vi "GetParamsVIS_K2182and6221.vi"(11 "KEITHLEY 2182 & KEITHLEY 6221_In":refnum<vi>) -> (0 "Params VIS K2182and6221_out":T2, 3 "KEITHLEY 2182 & KEITHLEY 6221_Out":refnum<vi>)   [LabVIEW 2013]
uses:
  TypeDef/EnumSelectedModeK2182and6221.ctl
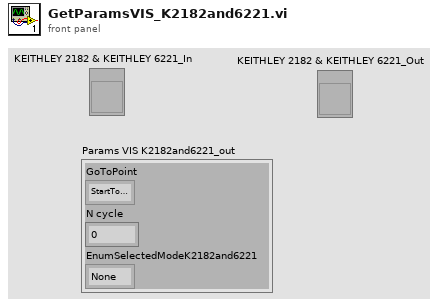
[diagram p1: front panel]
types:
  T1 = typedef "EnumSelectedModeK2182and6221.ctl" = enum16{"None", "K2182V", "K2182VI", "K2182VIS"}
  T2 = cluster{"GoToPoint":enum16{"StartToFront", "FrontToStart", "StartToBack", "BackToStart"}, "N cycle":i32, "EnumSelectedModeK2182and6221":T1}
  T3 = typedef "Keithly user program.lvlib/KE2182 -- Params.ctl" = cluster{"Auto Range?":bool, "Man / Selected\n       Range":enum16{"10mV", "100mV", "1V", "10V", "100V"}, "Enable Digital\n       Filter?":bool, "Filter Type":enum16{"Movin", "Repeat"}, "Filter Count":u32, "      Filter\nWindow (%)":dbl, "Enable Analog\n       Filter?":bool, "NPLCs":u32}
  T4 = typedef "Keithly user program.lvlib/KE622x -- Current Range.ctl" = cluster{"Auto Range?":bool, "Man / Selected\n        Range":enum16{"2nA", "20nA", "200nA", "2uA", "20uA", "200uA", "2mA", "20mA", "100mA"}}
  T5 = typedef "Keithly user program.lvlib/KE622x -- Current Level.ctl" = dbl
  T6 = typedef "Keithly user program.lvlib/KE622x -- Voltage Limit.ctl" = dbl
  T7 = typedef "Keithly user program.lvlib/KE6221 -- Output Response.ctl" = enum16{"Fast", "Slow"}
  T8 = cluster{"KEITHLEY ON/OFF":bool, "VISA KEITHLEY resource name":refnum<visa-resource-name>, "2182 -A Params":T3, "KEITHLEY CURRENT ON/OFF":bool, "6221 Params":cluster{"Current Range":T4, "Current Level (A)":T5, "Voltage Limit (V)":T6, "KE6221 Output Response":T7, "Analog Filter State":enum16{"Off", "On"}}, "Step Mode\nParams":bool, "Step Mode":cluster{"Front Point (A)":T5, "Start Point (A)":T5, "Back Point (A)":T5, "Step(A)":T5, "Time step (ms)":dbl, "N cycle":i32, "Sweeping":enum16{"Off Sweeping", "On Sweeping"}, "Go to":enum16{"Star Point", "Back Point"}}}
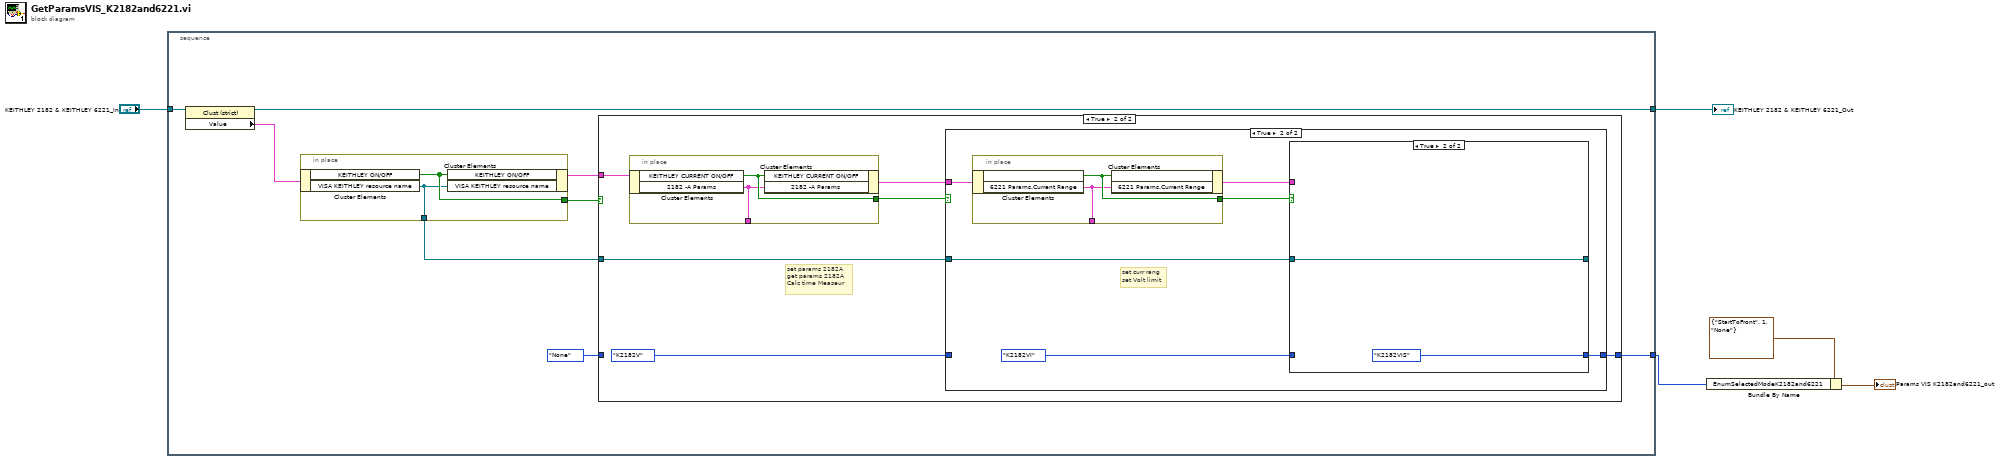
[diagram p0: block diagram]
diagram:
  n1 = stacked-sequence {
    tunnel: "KEITHLEY 2182 & KEITHLEY 6221_In" -> [w13]
    tunnel: [w12] -> w1
    tunnel: [w11] -> w5
    frame #0 {
      n2 = property class="Clust (strict)"(reference=w13) -> (reference out=w12:refnum<vi>, "Value"=w9:T8)  [unwired: 1 in, 1 out]
      n3 = in-place {
        in-place-border: [w15] -> w8
        in-place-border: [w14] -> w6
        n4 = in-place-cluster #1(w9) -> ("KEITHLEY ON/OFF"=w15:bool, "VISA KEITHLEY resource name"=w14:refnum<visa-resource-name>)
        n5 = in-place-cluster #1("KEITHLEY ON/OFF"=w15, "VISA KEITHLEY resource name"=w14) -> (w7:T8)
      }
      n6 = case shown="True" w8 {
        tunnel: w7 -> [_ w20]
        tunnel: [w16 w21] -> w11
        tunnel: EnumSelectedModeK2182and6221."None" -> [w16 _]
        tunnel: w6 -> [_ w17]
        frame False {
        }
        frame True {
          # "set params 2182A\nget params 2182A\nCalc time Measeur"
          n7 = in-place {
            in-place-border: [w24] -> w19
            in-place-border: [w23] -> _
            n8 = in-place-cluster #2(w20) -> ("KEITHLEY CURRENT ON/OFF"=w24:bool, "2182 -A Params"=w23:T3)
            n9 = in-place-cluster #2("KEITHLEY CURRENT ON/OFF"=w24, "2182 -A Params"=w23) -> (w18:T8)
          }
          n10 = case shown="True" w19 {
            tunnel: EnumSelectedModeK2182and6221."K2182V" -> [w25 _]
            tunnel: [w25 w30] -> w21
            tunnel: w18 -> [_ w28]
            tunnel: w17 -> [_ w29]
            frame False {
            }
            frame True {
              # "set curr rang\nset Volt limit"
              n11 = in-place {
                in-place-border: [w33] -> w27
                in-place-border: [w32] -> _
                n12 = in-place-cluster #3(w28) -> ("Step Mode\nParams"=w33:bool, "6221 Params.Current Range"=w32:T4)
                n13 = in-place-cluster #3("Step Mode\nParams"=w33, "6221 Params.Current Range"=w32) -> (w26:T8)
              }
              n14 = case shown="True" w27 {
                tunnel: EnumSelectedModeK2182and6221."K2182VI" -> [w35 _]
                tunnel: [w35 EnumSelectedModeK2182and6221."K2182VIS"] -> w30
                tunnel: w29 -> [w34 w36]
                tunnel: [w34 w36] -> _
                tunnel: w26 -> [_ _]
                frame False {
                  # "set curr level"
                }
                frame True {
                }
              }
            }
          }
        }
      }
    }
  }
  "KEITHLEY 2182 & KEITHLEY 6221_Out" <- w1
  n15 = Bundle By Name(cluster=T2 {"GoToPoint"=enum."StartToFront", "N cycle"=1, "EnumSelectedModeK2182and6221"=enum."None"}, "EnumSelectedModeK2182and6221"=w5) -> (→"Params VIS K2182and6221_out":T2)
